vi "errormessage.vi"(1 "error in":errorcluster) -> (0 "error out":errorcluster)   [LabVIEW 2013]
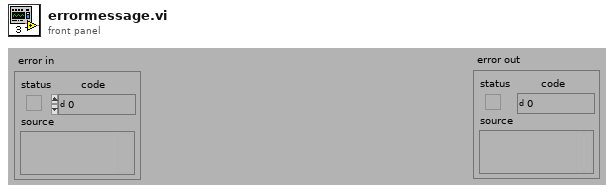
[diagram p1: front panel]
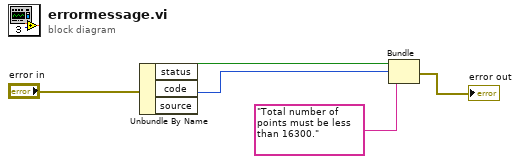
[diagram p0: block diagram]
diagram:
  n1 = Unbundle By Name("error in") -> ("status"=w4:bool, "code"=w3:i32)  [unwired: 1 out]
  n2 = Bundle("status"=w4, "code"=w3, "Total number of points must be less than 16300.") -> (→"error out":cluster{"status":bool, "code":i32, string})  [unwired: 1 in]
